vi "test Compile Driver Configuration.vi"(8 "error in (no error)":errorcluster, 11 "TestCase in":refnum<class "NI-SWITCH Compile Unit Tests.lvclass">) -> (0 "error out":errorcluster, 3 "TestCase out":refnum<class "NI-SWITCH Compile Unit Tests.lvclass">)   [LabVIEW 2017, in "NI-SWITCH Compile Unit Tests.lvclass"]
uses:
  NI-SWITCH Compile Unit Tests.lvclass
  Scripting/Properties/SLSC Switch All Properties.ctl
  Shared/Endpoint Configuration Cluster.ctl
  Shared/Endpoint Configuration Enum.ctl
  NI-SWITCH Compile Unit Tests.lvclass/NI-SWITCH Compile Unit Tests.ctl
  Scripting/Custom Device/Find All SLSC Switch Custom Devices.vi
  <vilib>/addons/_JKI Toolkits/VI Tester/TestCase.llb/TestCase.lvclass
  Scripting/NI-SWITCH Scripting.lvlib
  Shared/NI-SWITCH Shared.lvlib
  System Explorer/NI-SWITCH System Explorer.lvlib
  C:/Program Files (x86)/National Instruments/LabVIEW 2017/vi.lib/addons/_JKI Toolkits/VI Tester/TestCase.llb/TestCase.lvclass
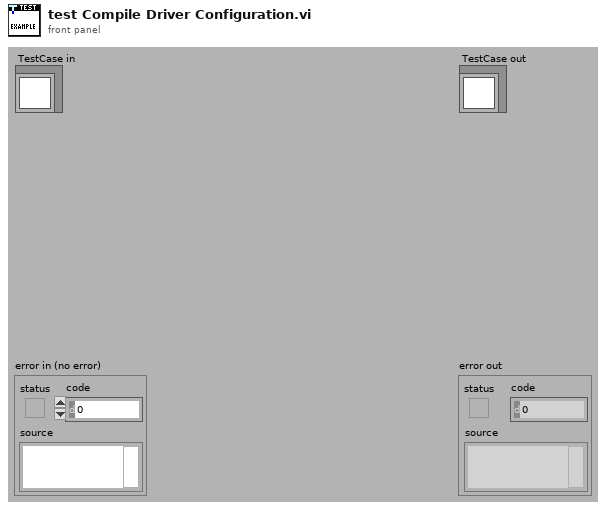
[diagram p1: front panel]
types:
  T1 = typedef "NI-SWITCH Scripting.lvlib/SLSC Switch All Properties.ctl" = cluster{"Product Name":string, "Topology":string, "Switches JSON":string, "Description":string, "Reservation Group":string}
  T2 = typedef "NI-SWITCH Shared.lvlib/Endpoint Configuration Cluster.ctl" = cluster{"Endpoint":string, "Configuration":T3}
  T3 = typedef "NI-SWITCH Shared.lvlib/Endpoint Configuration Enum.ctl" = enum16{"Load", "Source", "Configuration"}
  T4 = typedef "Custom Device API.lvlib/Custom Device Item Ref.ctl" = u64
  T5 = typedef "NI-SWITCH Shared.lvlib/Driver Configuration.ctl" = cluster{"Topology":string, "Switches JSON":string, "Source Channels":string[], "Configuration Channels":string[], "Reservation Group":string}
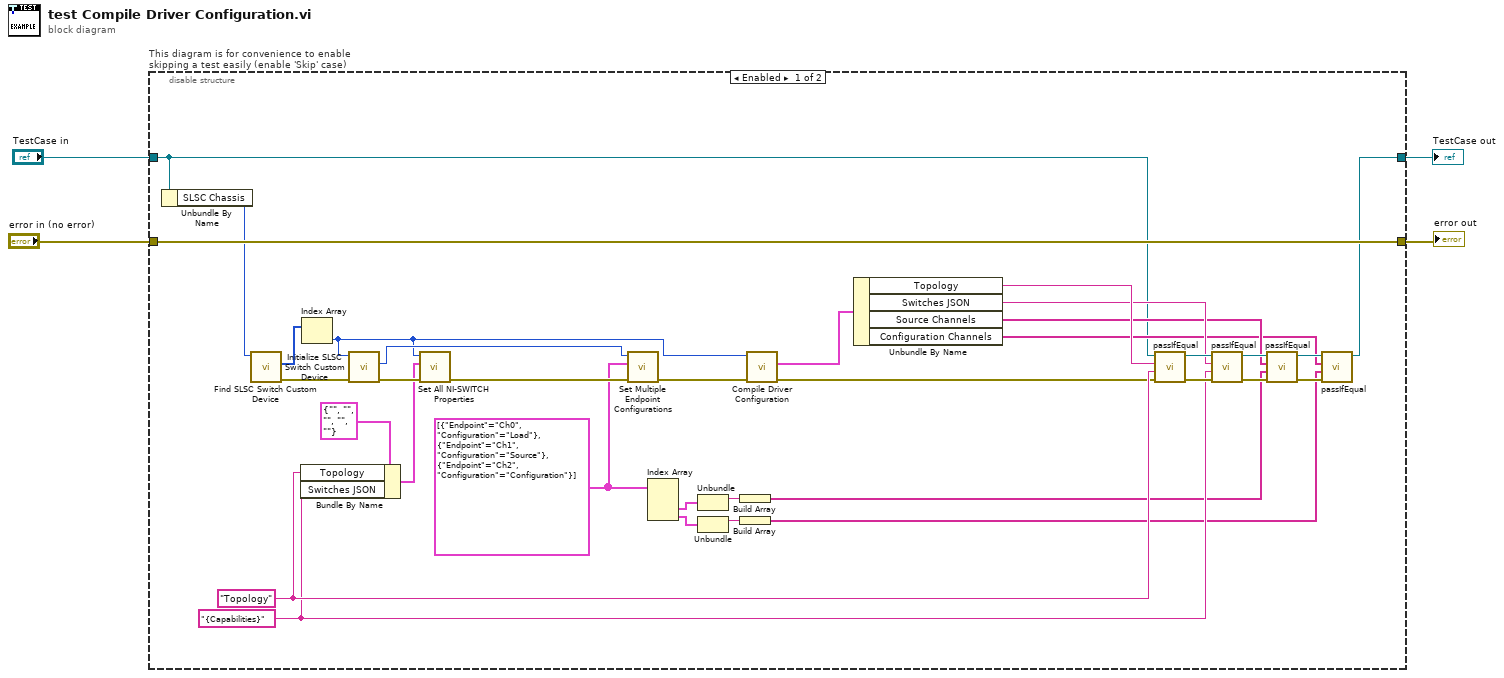
[diagram p0: block diagram]
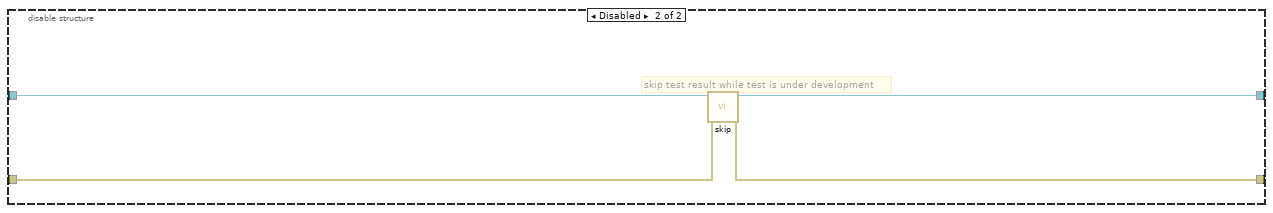
[diagram p2: hidden frame]
diagram:
  n1 = disable-structure "This diagram is for convenience to enable skipping a test easily (enable 'Skip' case)" shown="Enabled" {
    disable-tunnel: "TestCase in" -> [w8 w42]
    disable-tunnel: [w7 w40] -> w1
    disable-tunnel: [w38 w41] -> w3
    disable-tunnel: "error in (no error)" -> [w38 w39]
    frame Enabled {
      w22 = T2[] [{"Endpoint"="Ch0", "Configuration"=enum."Load"}, {"Endpoint"="Ch1", "Configuration"=enum."Source"}, {"Endpoint"="Ch2", "Configuration"=enum."Configuration"}] ("All Endpoint Configurations")
      w25 = "{Capabilities}" ("Capabilities")
      w29 = "Topology" ("Topology")
      n2 = Unbundle By Name(w8) -> ("SLSC Chassis"=w9:u64)
      n3 = call-poly "Find SLSC Switch Custom Device.vi"("slsc chassis in"=w9) -> ("error out"=w36:errorcluster, "ni-switch custom devices"=w37:T4[])  [unwired: 8 in, 1 out]
      n4 = Bundle By Name(cluster=T1 {"Product Name"="", "Topology"="", "Switches JSON"="", "Description"="", "Reservation Group"=""} ("SLSC Switch All Properties"), "Topology"=w29, "Switches JSON"=w25) -> (w33:T1)
      n5 = Index Array(array=w37) -> (element=w23:T4)  [unwired: 1 in]
      n6 = call "Initialize SLSC Switch Custom Device.vi"("error in"=w36, "ni-switch custom device in"=w23) -> ("error out"=w35:errorcluster, "endpoint configuration section"=w24:T4)  [unwired: 7 in, 1 out]
      n7 = call "Set All NI-SWITCH Properties.vi"("error in"=w35, "properties"=w33, "ni-switch custom device in"=w23) -> ("error out"=w32:errorcluster)  [unwired: 7 in, 1 out]
      n8 = call "Set Multiple Endpoint Configurations.vi"("error in"=w32, "endpoint configurations"=w22, "endpoint configuration in"=w24) -> ("error out"=w31:errorcluster)  [unwired: 7 in, 1 out]
      n9 = Index Array(array=w22) -> (element #2=w15:T2, element #3=w14:T2)  [unwired: 3 in, 1 out]
      n10 = Unbundle(w15) -> ("Endpoint"=w13:string)  [unwired: 1 out]
      n11 = Unbundle(w14) -> ("Endpoint"=w12:string)  [unwired: 1 out]
      n12 = Build Array(w13) -> (w11:string[])
      n13 = Build Array(w12) -> (w10:string[])
      n14 = call "Compile Driver Configuration.vi"("error in (no error)"=w31, "Device Ref in"=w23) -> ("error out"=w5:errorcluster, "Driver Configuration"=w6:T5)  [unwired: 7 in, 1 out]
      n15 = Unbundle By Name(w6) -> ("Topology"=w30:string, "Switches JSON"=w26:string, "Source Channels"=w19:string[], "Configuration Channels"=w16:string[])
      n16 = call-dynamic "passIfEqual.vi"("error in (no error)"=w5, "y"=w29, "x"=w30, "TestCase in"=w8) -> ("error out"=w28:errorcluster, "TestCase out"=w27:refnum<class "NI-SWITCH Compile Unit Tests.lvclass">)  [unwired: 6 in]
      n17 = call-dynamic "passIfEqual.vi"("error in (no error)"=w28, "y"=w25, "x"=w26, "TestCase in"=w27) -> ("error out"=w20:errorcluster, "TestCase out"=w21:refnum<class "NI-SWITCH Compile Unit Tests.lvclass">)  [unwired: 6 in]
      n18 = call-dynamic "passIfEqual.vi"("error in (no error)"=w20, "y"=w11, "x"=w19, "TestCase in"=w21) -> ("error out"=w17:errorcluster, "TestCase out"=w18:refnum<class "NI-SWITCH Compile Unit Tests.lvclass">)  [unwired: 6 in]
      n19 = call-dynamic "passIfEqual.vi"("error in (no error)"=w17, "y"=w10, "x"=w16, "TestCase in"=w18) -> ("TestCase out"=w7:refnum<class "NI-SWITCH Compile Unit Tests.lvclass">)  [unwired: 6 in, 1 out]
    }
    frame Disabled {
      # "skip test result while test is under development"
      n20 = call <vilib>:"skip.vi"("error in (no error)"=w39, "TestCase in"=w42) -> ("error out"=w41:errorcluster, "TestCase out"=w40:refnum<class "NI-SWITCH Compile Unit Tests.lvclass">)  [unwired: 8 in]
    }
  }
  "error out" <- w3
  "TestCase out" <- w1
